vi "获取默认流程路径.vi"(11 "参数":string[](array[string])) -> (3 "路径":path)   [LabVIEW 2016, in "斯坦道氨氮V2.lvlib"]
uses:
  <vilib>/Utility/sysdir.llb/System Directory Type.ctl
  <vilib>/regexp/Match Regular Expression.xnode
panel:
  out "正则表达式":string
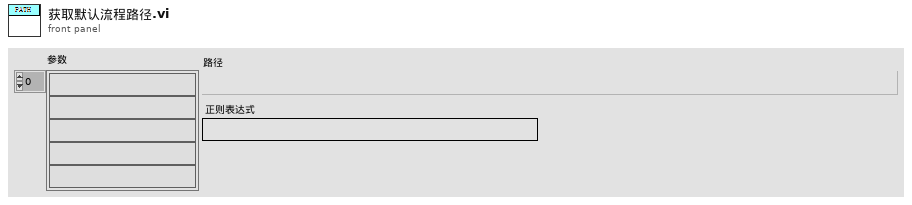
[diagram p1: front panel]
types:
  T1 = typedef "System Directory Type.ctl" = i32
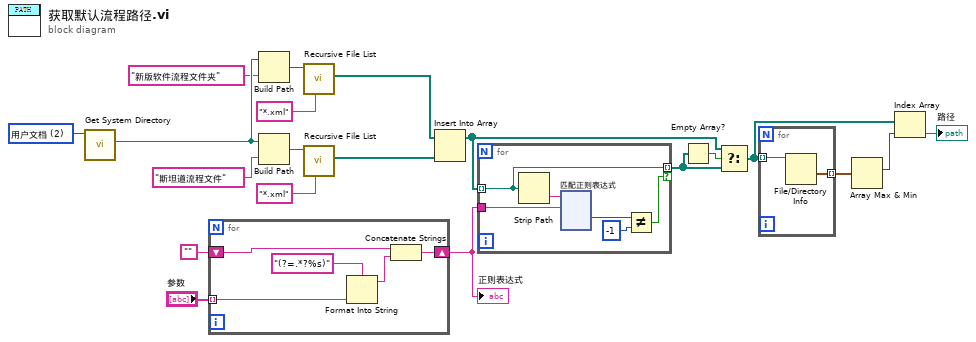
[diagram p0: block diagram]
diagram:
  w4 = T1 2 items=["用户目录"=0, "用户桌面"=1, "用户文档"=2, "用户应用程序数据"=3, "用户设置"=4, "用户临时目录"=5, "公共文档"=6, "公共应用程序数据"=7, "公共设置"=8, "公共缓存"=13, "系统核心库"=9, "系统安装库"=10, "应用程序文件"=11, "启动盘根目录"=12] ("system directory type")
  n1 = call <vilib>:"Get System Directory.vi"("system directory type"=w4) -> ("system directory"=w8:path)  [unwired: 10 in]
  n2 = for {
    tunnel: "参数" -> [w25] mode=indexing
    shift-right: [w22] -> w1
    shift-left: "" -> [w21]
    n3 = Format Into String(format string="(?=.*?%s)" ("格式字符串"), w25) -> (resulting string=w23:string)  [unwired: 2 in, 1 out]
    n4 = Concatenate Strings(w21, w23) -> (w22:string)
  }
  "正则表达式" <- w1
  n5 = Build Path(base path=w8, name or relative path="新版软件流程文件夹" ("名称或相对路径")) -> (appended path=w7:path)
  n6 = Build Path(base path=w8, name or relative path="斯坦道流程文件" ("名称或相对路径")) -> (appended path=w11:path)
  n7 = call <vilib>:"Recursive File List.vi"("pattern"="*.xml", "Folder Path"=w7) -> ("All Files in Dir"=w12:path[])  [unwired: 5 in, 4 out]
  n8 = call <vilib>:"Recursive File List.vi"("pattern"="*.xml", "Folder Path"=w11) -> ("All Files in Dir"=w13:path[])  [unwired: 5 in, 4 out]
  n9 = Insert Into Array(array=w12, new element=w13) -> (w18:path[])  [unwired: 1 in]
  n10 = for {
    tunnel: w18 -> [w29] mode=indexing
    tunnel: w1 -> [w30]
    tunnel: [w29] -> w19 mode=indexing if=w26
    n11 = Strip Path(path=w29) -> (name=w31:string)  [unwired: 1 out]
    n12 = xnode "匹配正则表达式"("输入字符串"=w31, "正则表达式"=w30) -> ("匹配后偏移量"=w28:i32)  [unwired: 4 in, 4 out]
    n13 = Not Equal?(x=w28, y=-1) -> (x != y?=w26:bool)
  }
  n14 = Empty Array?(array=w19) -> (empty?=w17:bool)
  n15 = Select(t=w18, s=w17, f=w19) -> (s? t:f=w20:path[])
  n16 = for {
    tunnel: w20 -> [w146] mode=indexing
    tunnel: [w147] -> w15 mode=indexing
    n17 = File/Directory Info(path=w146) -> (last mod=w147:timestamp)  [unwired: 1 in, 6 out]
  }
  n18 = Array Max & Min(array=w15) -> (max index (indices)=w14:i32)  [unwired: 3 out]
  n19 = Index Array(array=w20, index=w14) -> (element=→"路径":path)
